vi "FTW-System-CommandLineExecute.vi"(0 "Command":string, 5 "Standard Input":string, 7 "Working Directory":path, 9 "Blocking?":bool=TRUE, 11 "error in":errorcluster) -> (4 "Standard Output":string, 6 "Standard Error":string, 8 "Return Code":i32, 15 "error out":errorcluster)   [LabVIEW 2015]
panel:
  # "Inputs"
  # "Outputs"
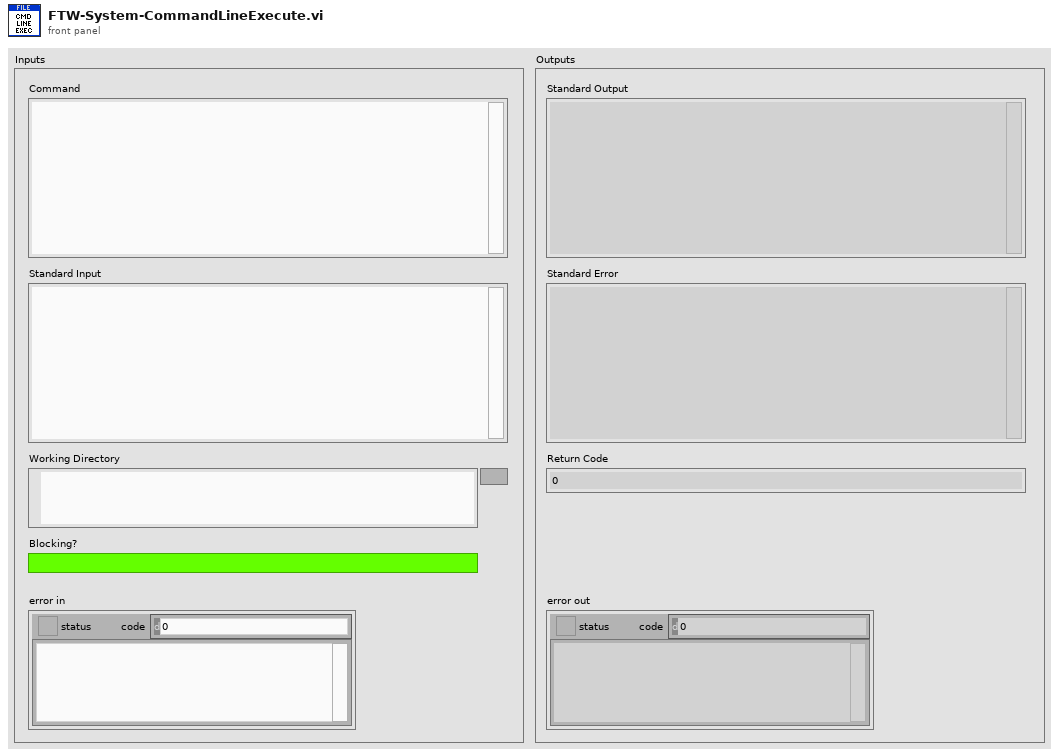
[diagram p1: front panel]
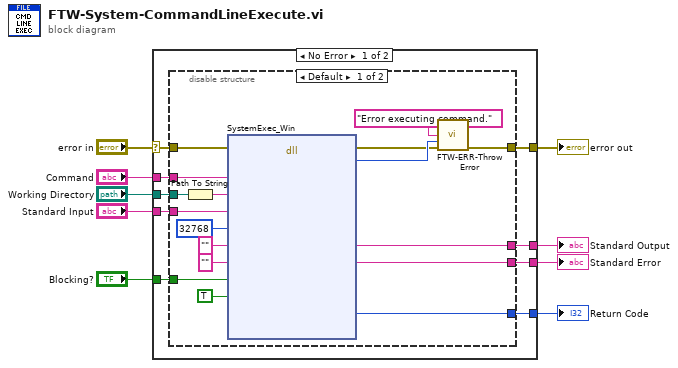
[diagram p0: block diagram]
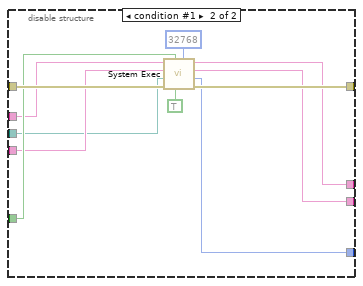
[diagram p2: hidden frame]
diagram:
  n1 = case shown="No Error" "error in" {
    selector: "error in" -> [w18 w47]
    tunnel: "Working Directory" -> [w16 _]
    tunnel: [w17 w47] -> w7
    tunnel: "Standard Input" -> [w15 _]
    tunnel: "Command" -> [w14 _]
    tunnel: [w13 _] -> w4
    tunnel: [w12 _] -> w3
    tunnel: [w11 _] -> w2
    tunnel: "Blocking?" -> [w10 _]
    frame No Error {
      n2 = disable-structure shown="Default" {
        disable-tunnel: w18 -> [w35 w46]
        disable-tunnel: [w29 w45] -> w17
        disable-tunnel: w16 -> [w28 w41]
        disable-tunnel: w15 -> [w27 w42]
        disable-tunnel: w14 -> [w26 w43]
        disable-tunnel: [w25 w38] -> w13
        disable-tunnel: [w24 w37] -> w12
        disable-tunnel: [w22 w36] -> w11
        disable-tunnel: w10 -> [w19 w44]
        frame condition #0 (active) {
          n3 = Path To String(path=w28) -> (string=w33:string)
          n4 = dll-call lib="LabVIEW" fn="SystemExec_Win"(error in=w35, "Command"=w26, "Working Directory"=w33, "Standard Input"=w27, "Expected Output Size"=u32 32768, "Standard Output"="", "Standard Error"="", "Blocking?"=w19, "Run Minimized"=TRUE) -> (error out=w30:errorcluster, "Return"=w32:i32, "Standard Output"=w25:string, "Standard Error"=w24:string, "Return Code"=w22:i32)  [unwired: 11 in, 1 out]
          n5 = call "FTW-ERR-ThrowError.vi"("Error Message"="Error executing command.", "Error Code"=w32, "error in"=w30) -> ("error out"=w29:errorcluster)  [unwired: 12 in]
        }
        frame condition #1 {
          n6 = call <vilib>:"System Exec.vi"("expected output size  (4096)"=u32 32768, "run minimized? (F)"=TRUE, "wait until completion? (T)"=w44, "error in (no error)"=w46, "working directory"=w41, "standard input"=w42, "command line"=w43) -> ("error out"=w45:errorcluster, "return code"=w36:i32, "standard error"=w37:string, "standard output"=w38:string)  [unwired: 1 in]
        }
      }
    }
    frame Error {
    }
  }
  "error out" <- w7
  "Standard Output" <- w4
  "Standard Error" <- w3
  "Return Code" <- w2
